vi "SDI Coordinate Straight Line Move.vi"() -> ()   [LabVIEW 2014]
uses:
  <vilib>/Motion/plugins/PluginFramework/nismSDIFramework.SetFrameworkMode.multi.vi
  <vilib>/Motion/Express/_s/nimc.ex.clearFaults.clearFaults.axis.vi
  <vilib>/Motion/Express/_s/nimc.ex.power.power.axis.vi
  <vilib>/Motion/Express/_s/nimc.ex.stopMove.stop.coordinate.modeDecelerate.vi
  <vilib>/Motion/Express/_s/nimc.ex.read.readExecutionData.coordinate.vi
  <vilib>/Motion/Express/_s/nimc.ex.straightLineMove.startStraightLineMove.coordinate.modeRelative.0.vi
  <vilib>/Motion/BlockNode/FB.NIMotion.xnode
  <vilib>/Motion/plugins/SDI Plug-in - Delta ASDA/Template SoftMotion Drive Interface Plug-in Class.lvclass
panel:
  in  "Y Axis":refnum<k21>="Axis 2"
  in  "X Axis":refnum<k21>="Axis 1"
  out "Move Done":bool
  out "Move Position":T1(graph)
  in  "X Pos":dbl=10000.0
  in  "Y Pos":dbl=7500.0
  in  "Velocity":dbl=1000.0
  in  "Resource":refnum<k21>="Coordinate Space 1"
  in  "Stop Move":bool
  out "error out":errorcluster
  out "Example Done":bool
  # "Move Constraints"
  # "Notes: \n1. This example uses preconfigured settings that may not be appropriate for your motion system. Review and update the axis settings using the Axis Configuration dialog box. Right-click each axis and select Properties to open the Axis Configuration dialog box. \n2. Running this example automatically activates all axes. Disable the \"Enable Drive on Transition to Active Mode\" option on the General Settings page of the Axis Configuration dialog box to prevent axes from activating when the VI runs.\n3. This example uses the default smoothing input to automatically calculate deceleration and jerk values. To specify these move constraints, create a control for the \"smoothing\" input.\n\nFor information about using this example in an actual motion system, refer to ni.com/info and enter Info Code nismex."
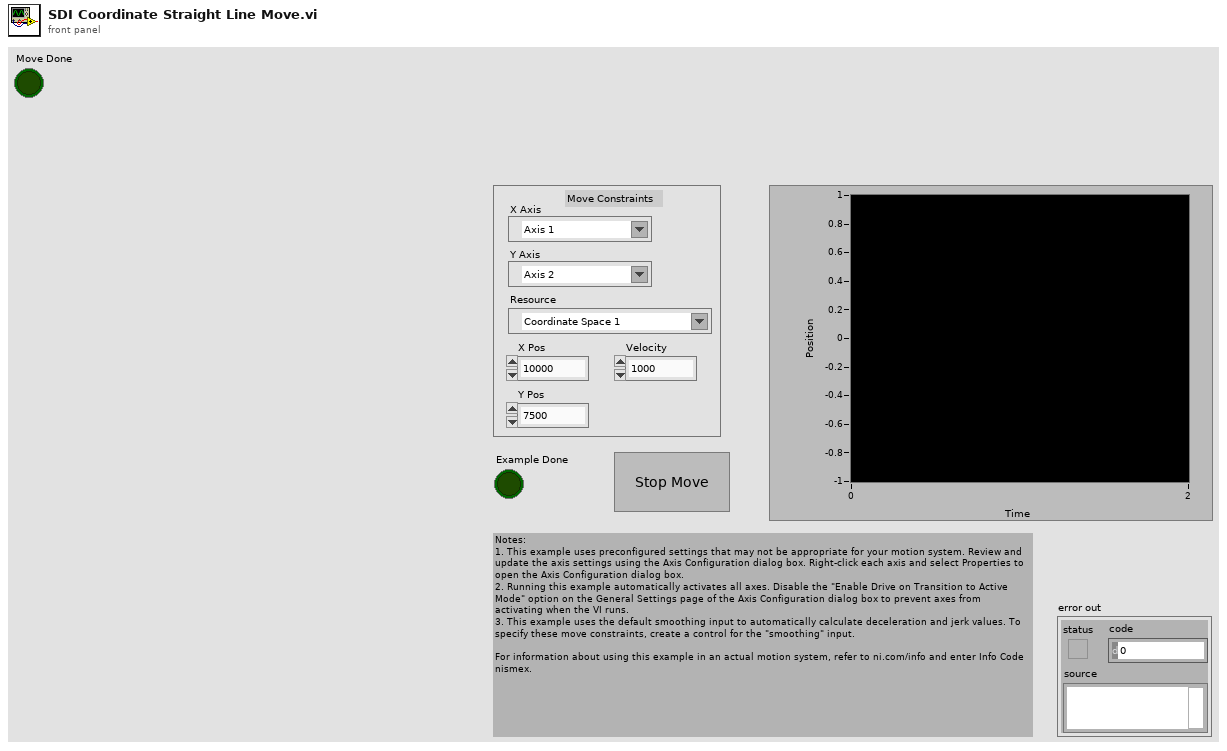
[diagram p1: front panel]
types:
  T1 = cluster{"position[] out[0]":dbl, "position[] out[1]":dbl, "position[] out[2]":dbl}
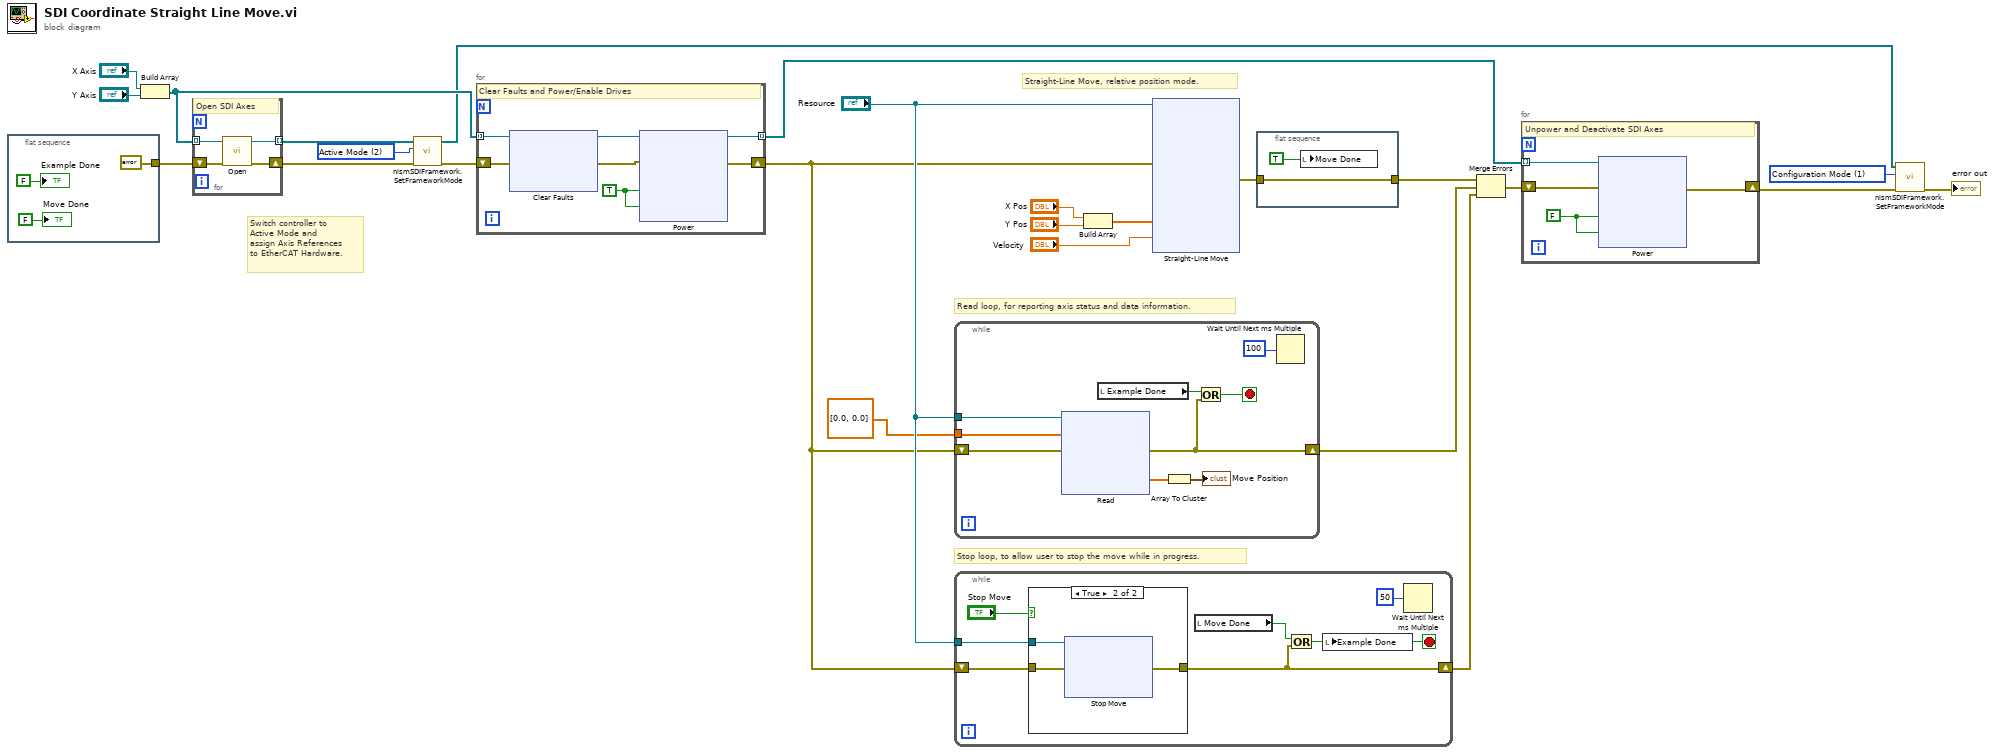
[diagram p0: block diagram]
diagram:
  w6 = 1 items=["Configuration Mode"=1, "Active Mode"=2] ("mode (Active Mode)")
  w16 = 2 items=["Configuration Mode"=1, "Active Mode"=2] ("mode (Active Mode)")
  # "Switch controller to\nActive Mode and \nassign Axis References\nto EtherCAT Hardware."
  # "Read loop, for reporting axis status and data information."
  # "Stop loop, to allow user to stop the move while in progress."
  # "Straight-Line Move, relative position mode."
  n1 = flat-sequence {
    tunnel: [w26] -> _
    tunnel: [w26] -> w7
    frame #0 {
      w26 = errorcluster {"status"=FALSE, "code"=0, "source"=""} ("Error")
      "Example Done" <- FALSE ("Example Done")
      "Move Done" <- FALSE ("Example Done")
    }
  }
  n2 = Build Array("X Axis", "Y Axis") -> (w12:refnum<k21>[])
  n3 = for {
    tunnel: w12 -> [w32] mode=indexing
    tunnel: [w31] -> w11 mode=indexing
    shift-right: [w30] -> w10
    shift-left: w7 -> [w29]
    # "Open SDI Axes"
    n4 = call <vilib>:"Open.vi"("error in (no error)"=w29, "Axis"=w32) -> ("error out"=w30:errorcluster, "Base Axis Out"=w31:refnum<class "nismPluginAxisBaseClass.lvclass">)  [unwired: 8 in]
  }
  n5 = call-poly <vilib>:"nismSDIFramework.SetFrameworkMode.vi"("error in (no error)"=w10, "mode (Active Mode)"=w16, "Base Axis In"=w11) -> ("error out"=w14:errorcluster, "Base Axis Out"=w1:refnum<class "nismPluginAxisBaseClass.lvclass">[])  [unwired: 7 in]
  n6 = for {
    tunnel: w12 -> [w35] mode=indexing
    tunnel: [w34] -> w2 mode=indexing
    shift-right: [w37] -> w9
    shift-left: w14 -> [w36]
    w39 = TRUE ("enable axis")
    # "Clear Faults and Power/Enable Drives"
    n7 = xnode ("Clear Faults")("resource"=w35, "error in"=w36) -> ("resource out"=w33:refnum<k21>, "error out"=w38:errorcluster)
    n8 = xnode ("Power")("enable axis"=w39, "enable drive"=w39, "resource"=w33, "error in"=w38) -> ("resource out"=w34:refnum<k21>, "error out"=w37:errorcluster)
  }
  n9 = while {
    tunnel: "Resource" -> [w60]
    tunnel: dbl[] [0.0, 0.0] -> [w54]
    shift-right: [w59] -> w25
    shift-left: w9 -> [w57]
    stop <- w62 stop-if-true
    n10 = xnode ("Read")("resource"=w60, "position[]"=w54, "error in"=w57) -> ("position[] out"=w56:dbl[], "error out"=w59:errorcluster)  [unwired: 3 out]
    n11 = local read "Example Done"() -> (w61:bool)
    n12 = Array To Cluster(array=w56) -> (cluster=→"Move Position":T1)
    n13 = Or(x=w61, y=w59) -> (x .or. y?=w62:bool)
    n14 = Wait Until Next ms Multiple(millisecond multiple=u32 100) -> ()  [unwired: 1 out]
  }
  n15 = while {
    tunnel: "Resource" -> [w75]
    shift-right: [w73] -> w24
    shift-left: w9 -> [w74]
    stop <- w71 stop-if-true
    n16 = case shown="True" "Stop Move" {
      tunnel: [w78 w81] -> w73
      tunnel: w75 -> [_ w80]
      tunnel: w74 -> [w78 w79]
      frame False {
      }
      frame True {
        n17 = xnode ("Stop Move")("resource"=w80, "error in"=w79) -> ("error out"=w81:errorcluster)  [unwired: 1 in, 2 out]
      }
    }
    n18 = local read "Move Done"() -> (w72:bool)
    n19 = Or(x=w72, y=w73) -> (x .or. y?=w71:bool)
    n20 = local write "Example Done"(w71) -> ()
    n21 = Wait Until Next ms Multiple(millisecond multiple=u32 50) -> ()  [unwired: 1 out]
  }
  n22 = Build Array("X Pos", "Y Pos") -> (w20:dbl[])
  n23 = xnode ("Straight-Line Move")("position[]"=w20, "velocity"="Velocity", "resource"="Resource", "error in"=w9) -> ("error out"=w17:errorcluster)  [unwired: 6 in, 2 out]
  n24 = flat-sequence {
    tunnel: w17 -> [w90]
    tunnel: [w90] -> w18
    frame #0 {
      n25 = local write "Move Done"(TRUE ("Example Done")) -> ()
    }
  }
  n26 = Merge Errors(w18, w25, w24) -> (w4:errorcluster)
  n27 = for {
    tunnel: w2 -> [w92] mode=indexing
    shift-right: [w94] -> w5
    shift-left: w4 -> [w93]
    w95 = FALSE ("enable axis")
    # "Unpower and Deactivate SDI Axes"
    n28 = xnode ("Power")("enable axis"=w95, "enable drive"=w95, "resource"=w92, "error in"=w93) -> ("error out"=w94:errorcluster)  [unwired: 1 out]
  }
  n29 = call-poly <vilib>:"nismSDIFramework.SetFrameworkMode.vi"("error in (no error)"=w5, "mode (Active Mode)"=w6, "Base Axis In"=w1) -> ("error out"=→"error out":errorcluster)  [unwired: 7 in, 1 out]
